vi "Lag Plot.vi"(8 "Lag":u32=1, 9 "Data array":dbl[](array[numeric]) format="%#.6g") -> (3 "Normal Probability Plot":cluster{"x":dbl, dbl}[](graph))   [LabVIEW 2023]
doc: "Plots a lag plot of the data. You can use this VI to plot simulated data if you want to experiment with lag plots."
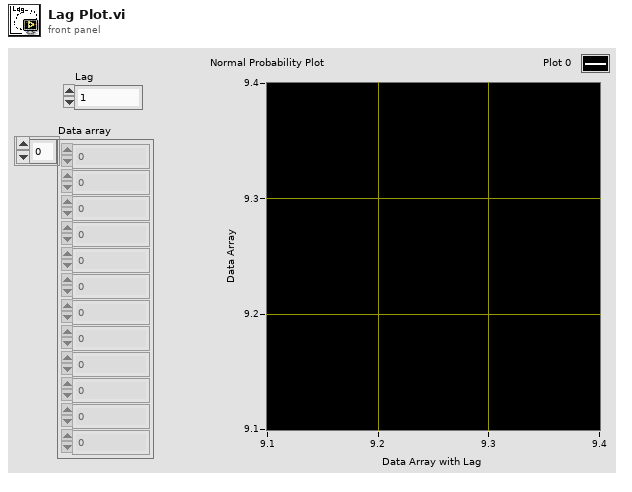
[diagram p1: front panel]
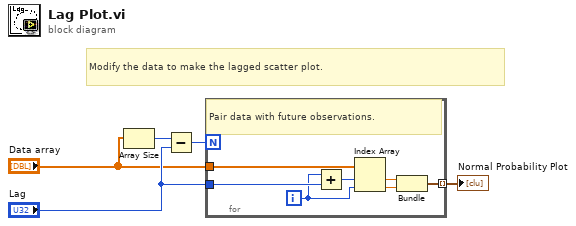
[diagram p0: block diagram]
diagram:
  # "Modify the data to make the lagged scatter plot."
  n1 = Array Size(array="Data array") -> (size(s)=w5:i32)
  n2 = Subtract(x=w5, y="Lag") -> (x-y=w4:u32)
  n3 = for {
    N: w4 -> [_]
    tunnel: "Lag" -> [w7]
    tunnel: "Data array" -> [w12]
    tunnel: [w8] -> w2 mode=indexing
    i -> [w6]
    # "Pair data with future observations."
    n4 = Add(x=w6, y=w7) -> (x+y=w11:u32)
    n5 = Index Array(array=w12, index #1=w11, index #2=w6) -> (element #1=w10:dbl, element #2=w9:dbl)
    n6 = Bundle(w10, w9) -> (w8:cluster{dbl, dbl})  [unwired: 1 in]
  }
  "Normal Probability Plot" <- w2
